vi "setOffset.vi"(8 "error in (no error)":errorcluster, 10 "Offset":dbl, 11 "VISA resource name":refnum<visa-resource-name>) -> (0 "error out":errorcluster, 3 "VISA resource name out":refnum<visa-resource-name>)   [LabVIEW 2023, in "Keysight-33500B.lvlib"]
doc: "<b>Author:</b> Wolfgang Rominger\n<b>Description:</b> >>>>Function converts the set input Frequency to a String in Scientific format and sends the FREQ commands >>>"
uses:
  Keysight-33500B.lvlib
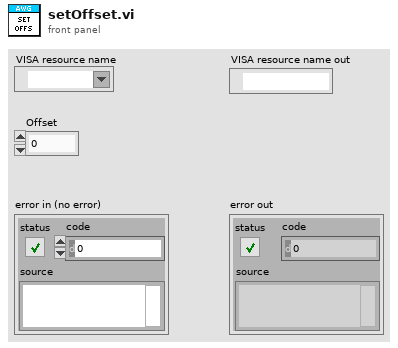
[diagram p1: front panel]
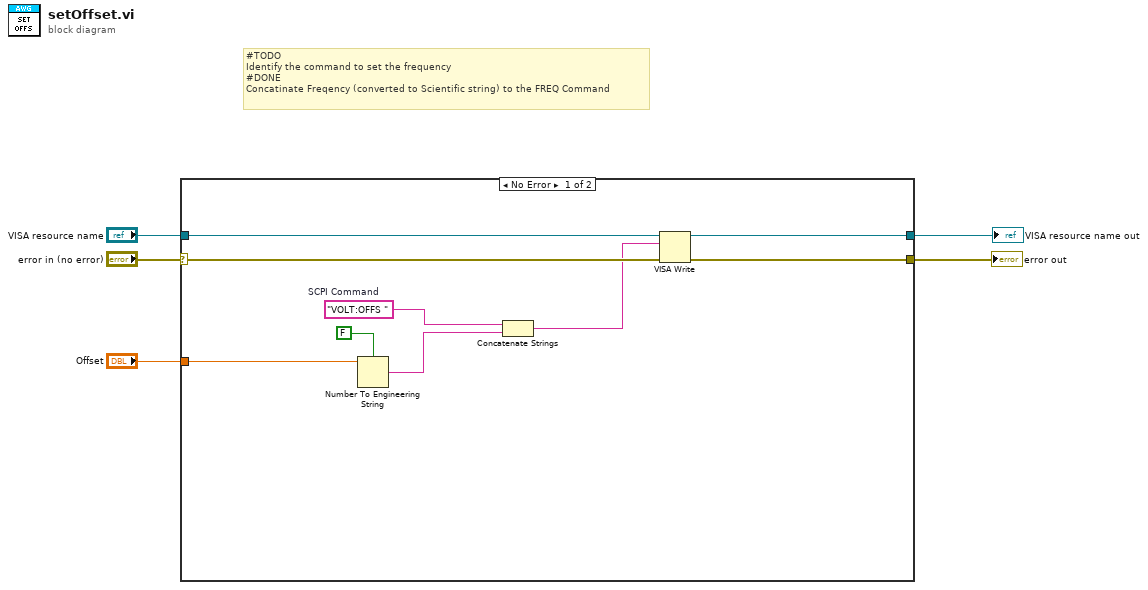
[diagram p0: block diagram]
diagram:
  # "#TODO\nIdentify the command to set the frequency\n#DONE\nConcatinate Freqency (converted to Scientific string) to the FREQ Command"
  n1 = case shown="No Error" "error in (no error)" {
    selector: "error in (no error)" -> [w13 w16]
    tunnel: [w7 w15] -> w5
    tunnel: [w8 w16] -> w3
    tunnel: "VISA resource name" -> [w14 w15]
    tunnel: "Offset" -> [w10 _]
    frame No Error {
      w12 = "VOLT:OFFS "  # SCPI Command
      n2 = Number To Engineering String(1:FALSE ("use system decimal point (T)"), 4:w10) -> (0:w9:string)  [unwired: 2 in]
      n3 = Concatenate Strings(w12, w9) -> (w11:string)
      n4 = VISA Write(VISA resource name=w14, write buffer=w11, error in (no error)=w13) -> (VISA resource name out=w7:refnum<visa-resource-name>, error out=w8:errorcluster)  [unwired: 1 out]
    }
    frame Error {
    }
  }
  "VISA resource name out" <- w5
  "error out" <- w3
